vi "SelectWallTrajectory.vi"(6 "Wall Position Limit":i32=360, 10 "New Wall Position":i32, 11 "Current Wall Position":dbl) -> (3 "StepSize":i32)   [LabVIEW 2013]
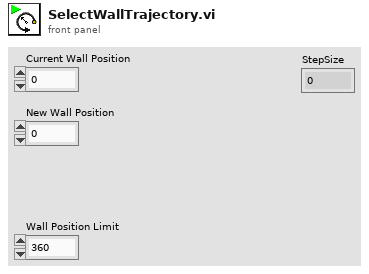
[diagram p1: front panel]
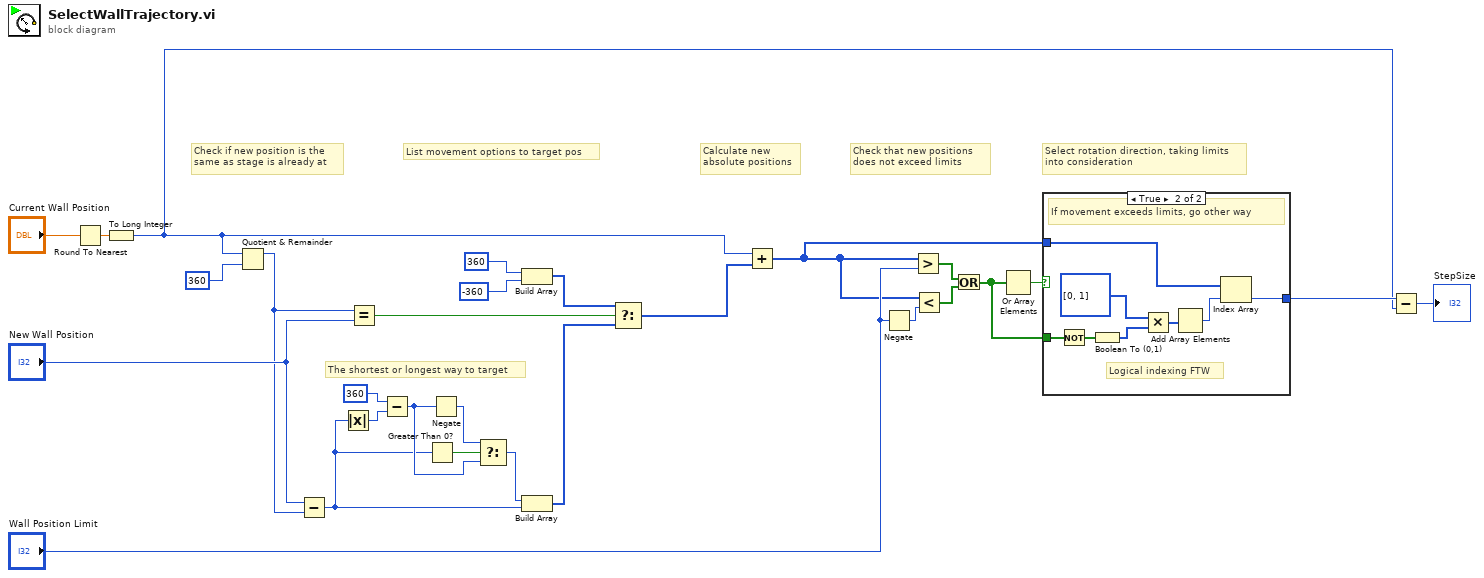
[diagram p0: block diagram]
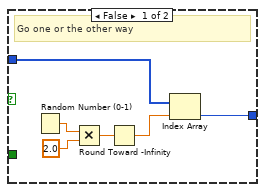
[diagram p2: hidden frame]
diagram:
  # "Calculate new \nabsolute positions"
  # "Select rotation direction, taking limits \ninto consideration"
  # "Check that new positions \ndoes not exceed limits"
  # "The shortest or longest way to target"
  # "List movement options to target pos"
  # "Check if new position is the \nsame as stage is already at"
  n1 = Round To Nearest(number="Current Wall Position") -> (nearest integer value=w27:dbl)
  n2 = To Long Integer(number=w27) -> (32bit integer=w2:i32)
  n3 = Quotient & Remainder(x=w2, y=360) -> (x-y*floor(x/y)=w20:i32)  [unwired: 1 out]
  n4 = Subtract(x="New Wall Position", y=w20) -> (x-y=w11:i32)
  n5 = Absolute Value(x=w11) -> (abs(x)=w17:i32)
  n6 = Equal?(x=w20, y="New Wall Position") -> (x = y?=w25:bool)
  n7 = Subtract(x=360, y=w17) -> (x-y=w15:i32)
  n8 = Greater Than 0?(x=w11) -> (x > 0?=w19:bool)
  n9 = Negate(x=w15) -> (-x=w16:i32)
  n10 = Select(t=w16, s=w19, f=w15) -> (s? t:f=w10:i32)
  n11 = Build Array(360 ("y"), -360 ("f")) -> (w12:i32[])
  n12 = Build Array(w10, w11) -> (w9:i32[])
  n13 = Select(t=w12, s=w25, f=w9) -> (s? t:f=w22:i32[])
  n14 = Add(x=w2, y=w22) -> (x+y=w8:i32[])
  n15 = Negate(x="Wall Position Limit") -> (-x=w23:i32)
  n16 = Greater?(x=w8, y="Wall Position Limit") -> (0:w7:bool[])
  n17 = Less?(x=w8, y=w23) -> (x < y?=w6:bool[])
  n18 = Or(x=w7, y=w6) -> (x .or. y?=w4:bool[])
  n19 = Or Array Elements(Boolean array=w4) -> (logical OR=w5:bool)
  n20 = case shown="True" w5 {
    tunnel: w8 -> [w31 w42]
    tunnel: w4 -> [_ w40]
    tunnel: [w29 w41] -> w3
    frame False {
      # "Go one or the other way"
      n21 = Random Number (0-1)() -> (number: 0 to 1=w34:dbl)
      n22 = Multiply(x=w34, y=2.0) -> (x*y=w32:dbl)
      n23 = Round Toward -Infinity(1:w32) -> (0:w30:dbl)
      n24 = Index Array(array=w31, index=w30) -> (element=w29:i32)
    }
    frame True {
      # "Logical indexing FTW"
      # "If movement exceeds limits, go other way"
      n25 = Not(x=w40) -> (.not. x?=w39:bool[])
      n26 = Boolean To (0,1)(Boolean=w39) -> (0, 1=w37:i16[])
      n27 = Multiply(x=i32[] [0, 1], y=w37) -> (x*y=w36:i32[])
      n28 = Add Array Elements(numeric array=w36) -> (sum=w35:i32)
      n29 = Index Array(array=w42, index=w35) -> (element=w41:i32)
    }
  }
  n30 = Subtract(x=w3, y=w2) -> (x-y=→"StepSize":i32)
